vi "Order Item Constructor.vi"(8 "error in (no error)":errorcluster, 9 "Cust Name":string, 10 "Pick Up Order Handler":refnum<class "Job Handler.lvclass">, 11 "Beverage":refnum<class "Beverage.lvclass">) -> (0 "error out":errorcluster, 3 "Order Item":refnum<class "Order Item.lvclass">)   [LabVIEW 2020, in "Order Item.lvclass"]
doc: "Package the beverage requested and the callback message to send upon completion as a new Order Item object."
uses:
  Order Item.lvclass
  Beverages/Beverage/Beverage.lvclass
  Order Item.lvclass/Order Item.ctl
  Process Job/Job Handler.lvclass
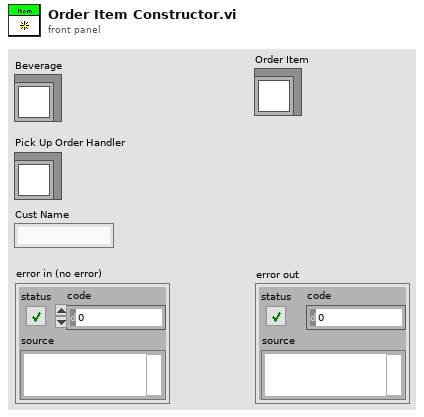
[diagram p1: front panel]
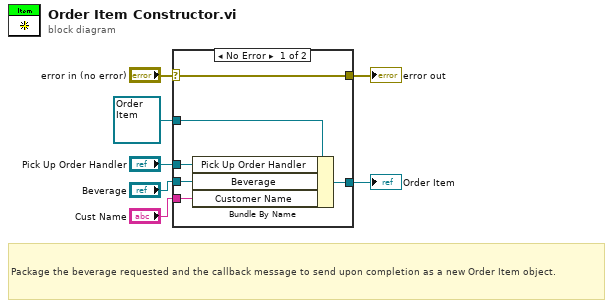
[diagram p0: block diagram]
diagram:
  # "Package the beverage requested and the callback message to send upon completion as a new Order Item object."
  n1 = case shown="No Error" "error in (no error)" {
    selector: "error in (no error)" -> [w11 w15]
    tunnel: [w11 w15] -> w6
    tunnel: refnum<class "Order Item.lvclass"> refnum ("Order Item.lvclass") -> [w13 w14]
    tunnel: [w12 w14] -> w4
    tunnel: "Beverage" -> [w10 _]
    tunnel: "Cust Name" -> [w9 _]
    tunnel: "Pick Up Order Handler" -> [w8 _]
    frame No Error {
      n2 = Bundle By Name(cluster=w13, "Pick Up Order Handler"=w8, "Beverage"=w10, "Customer Name"=w9) -> (w12:refnum<class "Order Item.lvclass">)
    }
    frame Error {
    }
  }
  "error out" <- w6
  "Order Item" <- w4
